vi "led_matr_v1.vi"() -> ()   [LabVIEW 2009]
panel:
  out "Coloana selectata":bool[](array[boolean])=[FALSE, TRUE, FALSE, TRUE, FALSE, FALSE, FALSE]
  in  "Array 3":bool[][](array[boolean])=[[FALSE, TRUE, TRUE, TRUE, FALSE], [TRUE, FALSE, FALSE, FALSE, TRUE], [FALSE, FALSE, FALSE, FALSE, TRUE], [FALSE, FALSE, TRUE, TRUE, FALSE], [FALSE, FALSE, FALSE, FALSE, TRUE], [TRUE, FALSE, FALSE, FALSE, TRUE], [FALSE, TRUE, TRUE, TRUE, FALSE]]
  in  "Coloana":u8(slide) scale=0.0..4.0
  in  "Iesire":bool
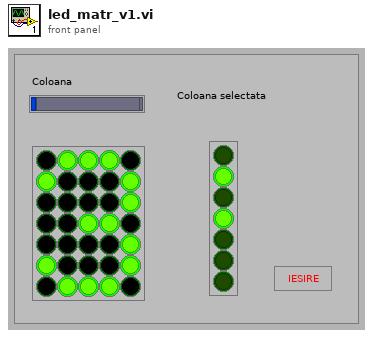
[diagram p1: front panel]
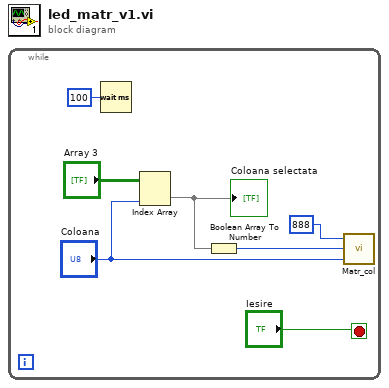
[diagram p0: block diagram]
diagram:
  n1 = while {
    stop <- "Iesire" stop-if-true
    n2 = Wait (ms)(milliseconds to wait=u32 100) -> ()  [unwired: 1 out]
    n3 = Index Array(array="Array 3", index (col)="Coloana") -> (element=w2:bool[])  [unwired: 1 in]
    "Coloana selectata" <- w2
    n4 = Boolean Array To Number(Boolean array=w2) -> (number=w1:u32)
    n5 = call "Matr_col.vi"("Coloana"="Coloana", "Date"=w1, "Adresa"=u32 888 ("milliseconds to wait")) -> ()  [unwired: 2 out]
  }
